vi "LVClasse_Surface Read Surface.vi"(8 "error in (no error)":errorcluster, 11 "Surface in":refnum<class "Surface.lvclass">) -> (0 "error out":errorcluster, 2 "Surface":i32, 3 "Surface out":refnum<class "Surface.lvclass">)   [LabVIEW 2020, in "Surface.lvclass"]
uses:
  Surface.lvclass
  Surface.lvclass/Surface.ctl
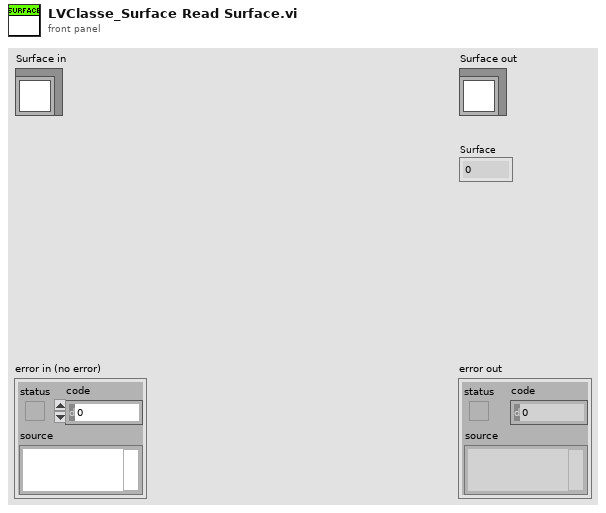
[diagram p1: front panel]
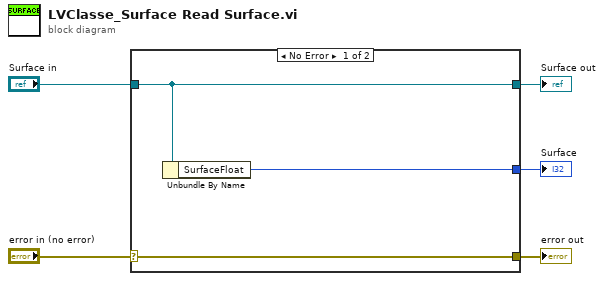
[diagram p0: block diagram]
diagram:
  n1 = case shown="No Error" "error in (no error)" {
    selector: "error in (no error)" -> [w8 w9]
    tunnel: [w8 w9] -> w4
    tunnel: [w7 w10] -> w2
    tunnel: "Surface in" -> [w7 w10]
    tunnel: [w6 _] -> w1
    frame No Error {
      n2 = Unbundle By Name(w7) -> ("SurfaceFloat"=w6:i32)
    }
    frame Error {
    }
  }
  "error out" <- w4
  "Surface out" <- w2
  "Surface" <- w1
